vi "GFG wait for variable.vi"(9 "Variant":variant, 10 "Variable Name":string, 11 "Source VI":string) -> ()   [LabVIEW 2012, in "GFG library.lvlib"]
uses:
  GFG library.lvlib
panel:
  out "error out":errorcluster
  in  "error in (no error)":errorcluster
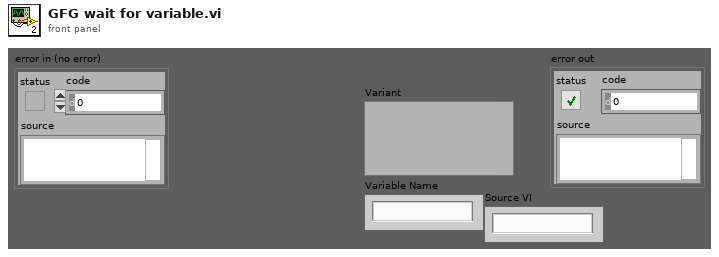
[diagram p1: front panel]
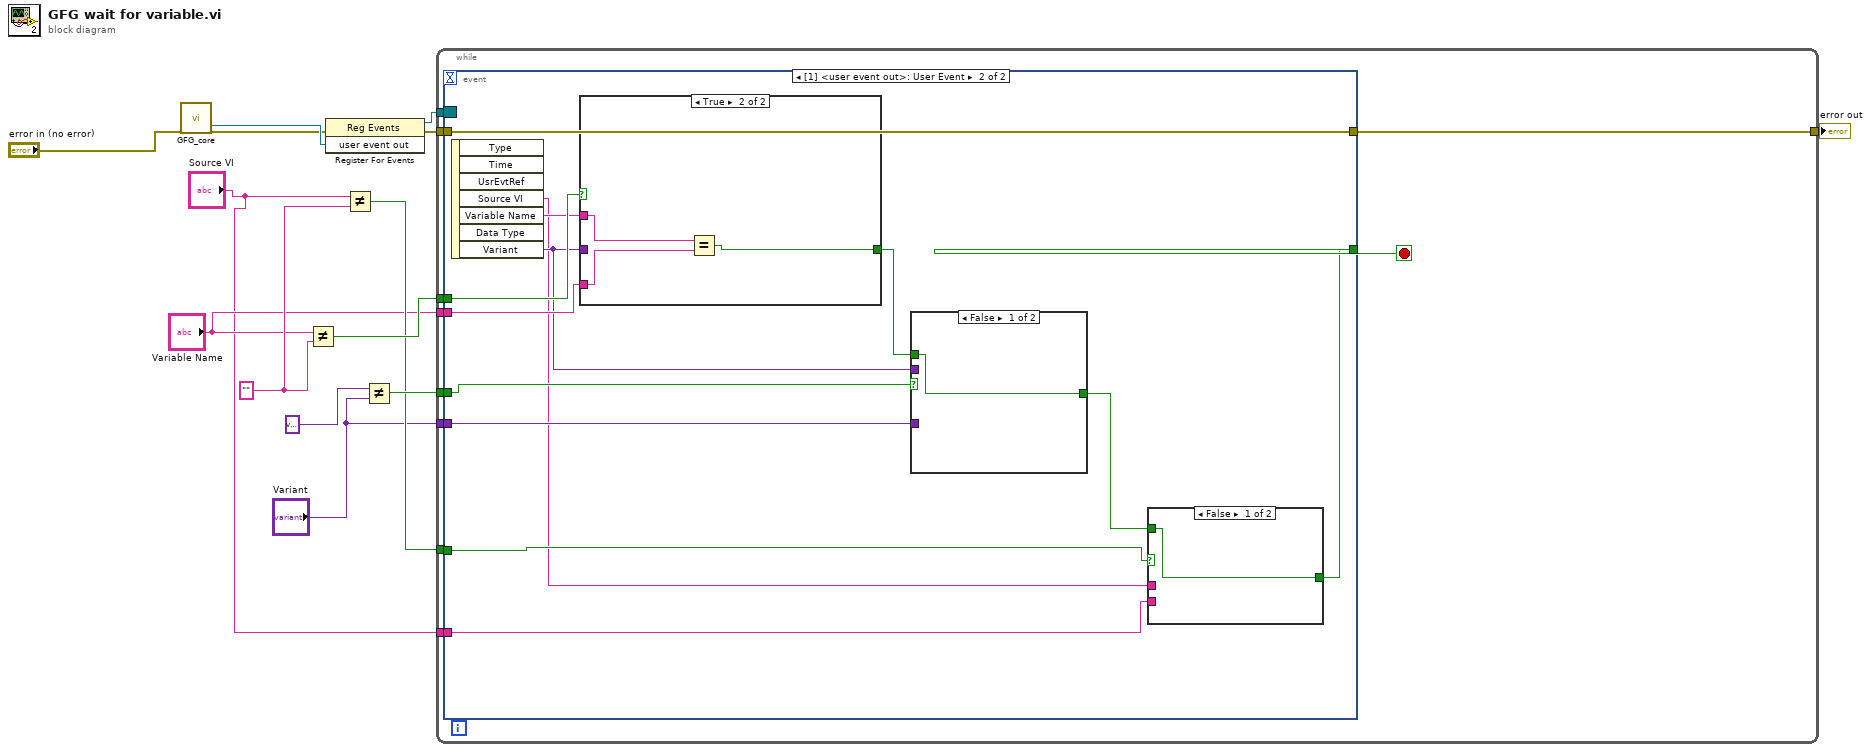
[diagram p0: block diagram]
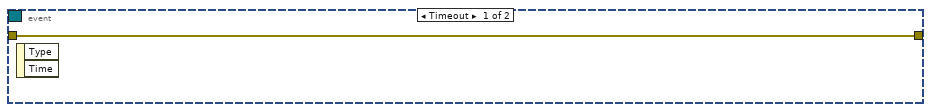
[diagram p2: hidden frame]
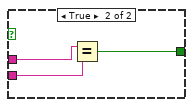
[diagram p3: hidden frame]
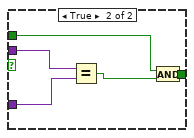
[diagram p4: hidden frame]
diagram:
  w6 = "" ("Variable Name")
  n1 = call "GFG_core.vi"("error in (no error)"="error in (no error)") -> ("user event out"=w13:refnum<user-event>, "error out"=w12:errorcluster)  [unwired: 12 in, 5 out]
  n2 = Not Equal?(x="Variable Name", y=w6) -> (x != y?=w7:bool)
  n3 = register-events(error in=w12, w13) -> (reference out=w14:refnum<event-registration>, error out=w10:errorcluster)  [unwired: 1 in]
  n4 = Not Equal?(x="Source VI", y=w6) -> (x != y?=w4:bool)
  n5 = Not Equal?(x=variant ("Variant"), y="Variant") -> (x != y?=w5:bool)
  n6 = while {
    tunnel: w14 -> [w24]
    tunnel: w10 -> [w22]
    tunnel: [w21] -> w9
    tunnel: w7 -> [w20]
    tunnel: w5 -> [w19]
    tunnel: w4 -> [w18]
    tunnel: "Variable Name" -> [w17]
    tunnel: "Variant" -> [w16]
    tunnel: "Source VI" -> [w15]
    stop <- w23 stop-if-true
    n7 = event shown="[1] <user event out>: User Event" {
      selector: w24 -> [_ _]
      dyn-events: _ -> [_ _]
      timeout: _ -> [_ _]
      tunnel: [_ w26] -> w23
      tunnel: w22 -> [w25 w38]
      tunnel: [w25 w38] -> w21
      tunnel: w20 -> [_ w37]
      tunnel: w19 -> [_ w33]
      tunnel: w18 -> [_ w30]
      tunnel: w17 -> [_ w35]
      tunnel: w16 -> [_ w31]
      tunnel: w15 -> [_ w28]
      event Timeout {
        n8 = event-data() -> ()  [unwired: 1 in, 2 out]
      }
      event User Event {
        n9 = event-data() -> ("Source VI"=w27:string, "Variable Name"=w36:string, "Variant"=w32:variant)  [unwired: 1 in, 4 out]
        n10 = case shown="True" w37 {
          tunnel: w36 -> [_ w51]
          tunnel: w32 -> [_ _]
          tunnel: [_ w49] -> w34
          tunnel: w35 -> [_ w50]
          frame False {
          }
          frame True {
            n11 = Equal?(x=w51, y=w50) -> (x = y?=w49:bool)
          }
        }
        n12 = case shown="False" w33 {
          tunnel: w34 -> [w43 w45]
          tunnel: w32 -> [_ w48]
          tunnel: w31 -> [_ w47]
          tunnel: [w43 w44] -> w29
          frame False {
          }
          frame True {
            n13 = Equal?(x=w48, y=w47) -> (x = y?=w46:bool)
            n14 = And(x=w45, y=w46) -> (x .and. y?=w44:bool)
          }
        }
        n15 = case shown="False" w30 {
          tunnel: w29 -> [w39 _]
          tunnel: w28 -> [_ w41]
          tunnel: w27 -> [_ w42]
          tunnel: [w39 w40] -> w26
          frame False {
          }
          frame True {
            n16 = Equal?(x=w42, y=w41) -> (x = y?=w40:bool)
          }
        }
      }
    }
  }
  "error out" <- w9
